vi "Set Sender.vi"(10 "Sender":refnum<class "Sender.lvclass">, 11 "Teardown Msg Strategy in":refnum<class "Teardown Msg Strategy.lvclass">) -> (3 "Teardown Msg Strategy out":refnum<class "Teardown Msg Strategy.lvclass">)   [LabVIEW 2021, in "Teardown Msg Strategy.lvlib" / "Teardown Msg Strategy.lvclass"]
uses:
  Teardown Msg Strategy.lvclass
  Teardown Msg Strategy.lvclass/Teardown Msg Strategy.ctl
  jettl/Sender/Sender/Sender.lvclass
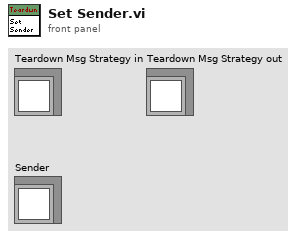
[diagram p1: front panel]
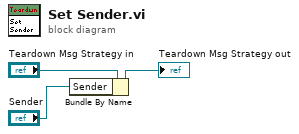
[diagram p0: block diagram]
diagram:
  n1 = Bundle By Name(cluster="Teardown Msg Strategy in", "Sender"="Sender") -> (→"Teardown Msg Strategy out":refnum<class "Teardown Msg Strategy.lvclass">)
